vi "VBus to Relay.vi"(2 "Invert Relay? (F)":bool, 3 "Motor VBus":dbl) -> (0 "RelayValue":T1)   [LabVIEW 2012]
uses:
  <vilib>/Rock Robotics/WPI/Relay/WPI_RelayValue.ctl
panel:
  # "Gets a VBus value and converts it to work with a Relay."
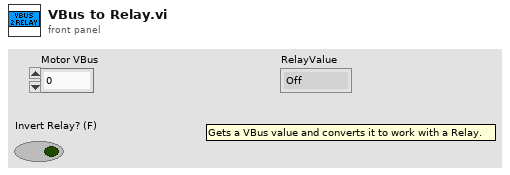
[diagram p1: front panel]
types:
  T1 = typedef "WPI_RelayValue.ctl" = enum16{"Off", "On", "Forward", "Reverse"}
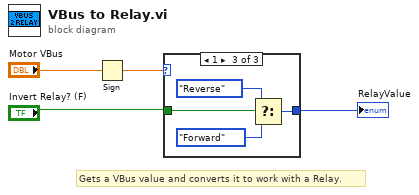
[diagram p0: block diagram]
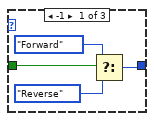
[diagram p2: hidden frame]
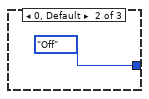
[diagram p3: hidden frame]
diagram:
  # "Gets a VBus value and converts it to work with a Relay."
  n1 = Sign(1:"Motor VBus") -> (0:w4:dbl)
  n2 = case shown="1" w4 {
    tunnel: [w5 WPI_RelayValue."Off" ("RelayValue") w12] -> w2
    tunnel: "Invert Relay? (F)" -> [w6 _ w13]
    frame -1 {
      n3 = Select(t=WPI_RelayValue."Forward" ("RelayValue"), s=w6, f=WPI_RelayValue."Reverse" ("RelayValue")) -> (s? t:f=w5:T1)
    }
    frame 0, Default {
    }
    frame 1 {
      n4 = Select(t=WPI_RelayValue."Reverse" ("RelayValue"), s=w13, f=WPI_RelayValue."Forward" ("RelayValue")) -> (s? t:f=w12:T1)
    }
  }
  "RelayValue" <- w2
